vi "output.vi"(8 "error in":errorcluster, 10 "data table in":T1, 11 "OPC UA runtime in":refnum<class "OPC UA Client runtime.lvclass">) -> (0 "error out":errorcluster, 2 "data table out":T1, 3 "OPC UA runtime out":refnum<class "OPC UA Client runtime.lvclass">)   [LabVIEW 2014, in "OPC UA Client runtime.lvclass"]
doc: "Provides an interface for writing data to a module at runtime. While this interface performs no operations, a child should provide an override which may write to any open sessions, references, or interfaces."
uses:
  OPC UA Client runtime.lvclass
  <vilib>/NI/Tag Bus/table/data table.ctl
  OPC UA Client runtime.lvclass/OPC UA Client runtime.ctl
  <vilib>/NI/Tag Bus/table/data polymorphs/read one/read Boolean.vi
  <vilib>/NI/Tag Bus/table/data polymorphs/read one/read I8.vi
  <vilib>/NI/Tag Bus/table/data polymorphs/read one/read U8.vi
  <vilib>/NI/Tag Bus/table/data polymorphs/read one/read I16.vi
  <vilib>/NI/Tag Bus/table/data polymorphs/read one/read U16.vi
  <vilib>/NI/Tag Bus/table/data polymorphs/read one/read I32.vi
  <vilib>/NI/Tag Bus/table/data polymorphs/read one/read U32.vi
  <vilib>/NI/Tag Bus/table/data polymorphs/read one/read I64.vi
  <vilib>/NI/Tag Bus/table/data polymorphs/read one/read U64.vi
  <vilib>/NI/Tag Bus/table/data polymorphs/read one/read Single.vi
  <vilib>/NI/Tag Bus/table/data polymorphs/read one/read Double.vi
  <vilib>/NI/Tag Bus/table/data polymorphs/read one/read String.vi
  <vilib>/NI/Tag Bus/table/data polymorphs/read one/read Array of Boolean.vi
  <vilib>/NI/Tag Bus/table/data polymorphs/read one/read Array of I8.vi
  <vilib>/NI/Tag Bus/table/data polymorphs/read one/read Array of U8.vi
  <vilib>/NI/Tag Bus/table/data polymorphs/read one/read Array of I16.vi
  <vilib>/NI/Tag Bus/table/data polymorphs/read one/read Array of U16.vi
  <vilib>/NI/Tag Bus/table/data polymorphs/read one/read Array of I32.vi
  <vilib>/NI/Tag Bus/table/data polymorphs/read one/read Array of U32.vi
  <vilib>/NI/Tag Bus/table/data polymorphs/read one/read Array of I64.vi
  <vilib>/NI/Tag Bus/table/data polymorphs/read one/read Array of U64.vi
  <vilib>/NI/Tag Bus/table/data polymorphs/read one/read Array of Single.vi
  <vilib>/NI/Tag Bus/table/data polymorphs/read one/read Array of Double.vi
  <vilib>/NI/Tag Bus/table/data polymorphs/read one/read Array of String.vi
  <vilib>/OPCUA/client/Write Bool.vi
  <vilib>/OPCUA/client/Write SByte.vi
  <vilib>/OPCUA/client/Write Byte.vi
  <vilib>/OPCUA/client/Write Int16.vi
  <vilib>/OPCUA/client/Write UInt16.vi
  <vilib>/OPCUA/client/Write Int32.vi
  <vilib>/OPCUA/client/Write UInt32.vi
  <vilib>/OPCUA/client/Write Int64.vi
  <vilib>/OPCUA/client/Write UInt64.vi
  <vilib>/OPCUA/client/Write Float.vi
  <vilib>/OPCUA/client/Write Double.vi
  <vilib>/OPCUA/client/Write String.vi
  <vilib>/OPCUA/client/Write DateTime.vi
  <vilib>/OPCUA/client/Write ByteString.vi
  <vilib>/OPCUA/client/Write Bool Array.vi
  <vilib>/OPCUA/client/Write SByte Array.vi
  <vilib>/OPCUA/client/Write Byte Array.vi
  <vilib>/OPCUA/client/Write Int16 Array.vi
  <vilib>/OPCUA/client/Write UInt16 Array.vi
  <vilib>/OPCUA/client/Write Int32 Array.vi
  <vilib>/OPCUA/client/Write UInt32 Array.vi
  <vilib>/OPCUA/client/Write Int64 Array.vi
  <vilib>/OPCUA/client/Write UInt64 Array.vi
  <vilib>/OPCUA/client/Write Float Array.vi
  <vilib>/OPCUA/client/Write Double Array.vi
  <vilib>/OPCUA/client/Write String Array.vi
  <vilib>/OPCUA/client/Write DateTime Array.vi
  <vilib>/OPCUA/client/Write ByteString Array.vi
  <vilib>/Utility/error.llb/Error Cluster From Error Code.vi
  <vilib>/ErrorRing/Error Ring.xnode
  <vilib>/NI/Tag Bus/table/data table.lvlib
  <vilib>/OPCUA/NI OPC UA Client.lvlib
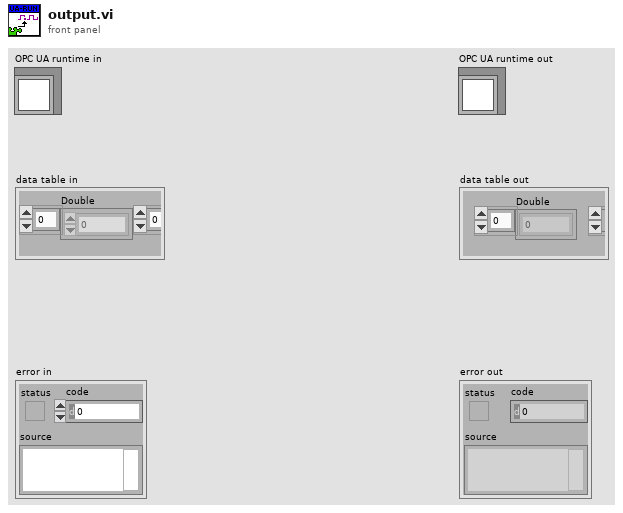
[diagram p1: front panel]
types:
  T1 = typedef "tag bus.lvlib/data table.lvlib/data table.ctl" = cluster{"Double":dbl[], "Single":sgl[], "I64":i64[], "I32":i32[], "I16":i16[], "I8":i8[], "U64":u64[], "U32":u32[], "U16":u16[], "U8":u8[], "Boolean":bool[], "String":string[], "Array of Double":cluster{"DBL Array":dbl[]}[], "Array of Single":cluster{"SGL Array":sgl[]}[], "Array of I64":cluster{"I64 Array":i64[]}[], "Array of I32":cluster{"I32 Array":i32[]}[], "Array of I16":cluster{"I16 Array":i16[]}[], "Array of I8":cluster{"I8 Array":i8[]}[], "Array of U64":cluster{"U64 Array":u64[]}[], "Array of U32":cluster{"U32 Array":u32[]}[], "Array of U16":cluster{"U16 Array":u16[]}[], "Array of U8":cluster{"U8 Array":u8[]}[], "Array of Boolean":cluster{"Boolean Array":bool[]}[], "Array of String":cluster{"String Array":string[]}[]}
  T2 = typedef "tag bus.lvlib/tag descriptor.lvclass/Data Type.ctl" = enum16{"Double", "Single", "I64", "I32", "I16", "I8", "U64", "U32", "U16", "U8", "Boolean", "String", "Array of Double", "Array of Single", "Array of I64", "Array of I32", "Array of I16", "Array of I8", "Array of U64", "Array of U32", "Array of U16", "Array of U8", "Array of Boolean", "Array of String"}
  T3 = typedef "OPC UA Client configuration.lvclass/OPC UA Data Type.ctl" = u16
  T4 = cluster{"DCAF Data Type":T2, "Index":i32, "Node Path":string, "OPC UA Data Type":T3}[]
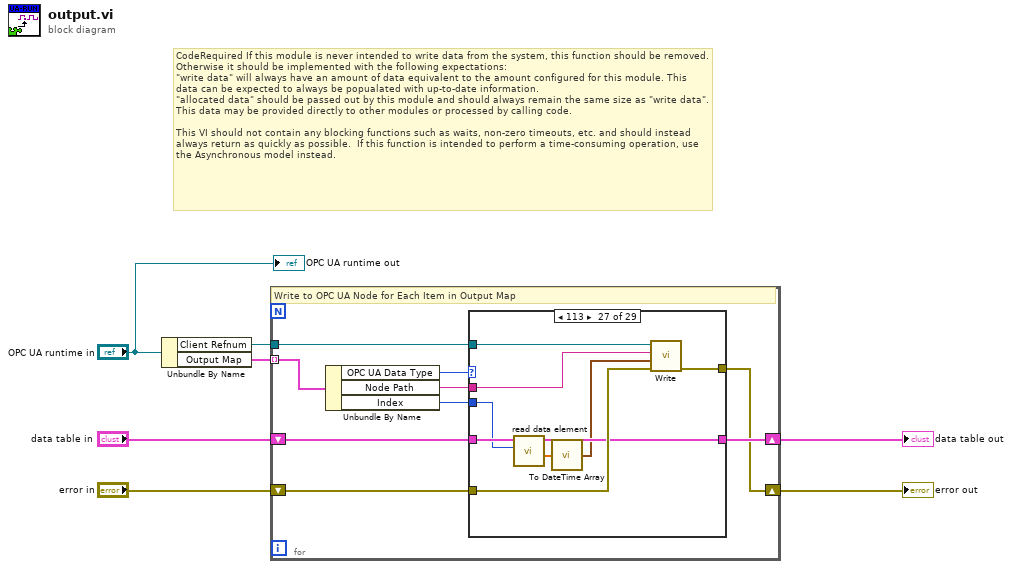
[diagram p0: block diagram]
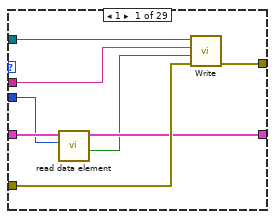
[diagram p2: hidden frame]
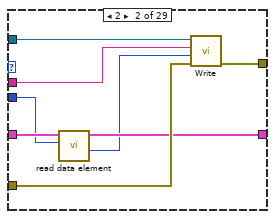
[diagram p3: hidden frame]
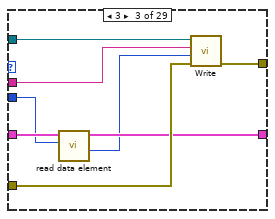
[diagram p4: hidden frame]
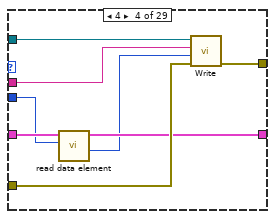
[diagram p5: hidden frame]
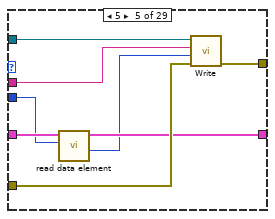
[diagram p6: hidden frame]
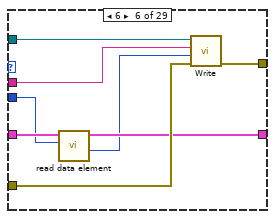
[diagram p7: hidden frame]
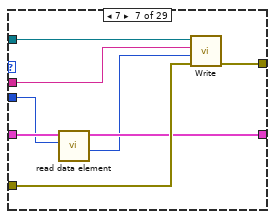
[diagram p8: hidden frame]
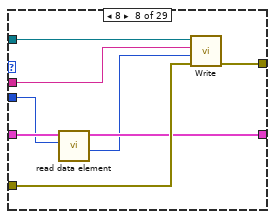
[diagram p9: hidden frame]
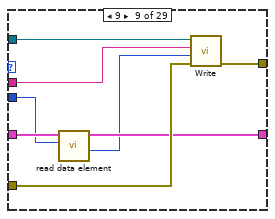
[diagram p10: hidden frame]
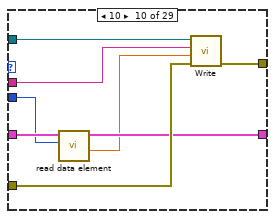
[diagram p11: hidden frame]
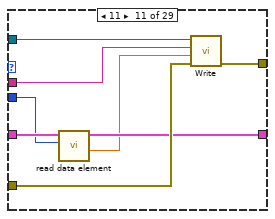
[diagram p12: hidden frame]
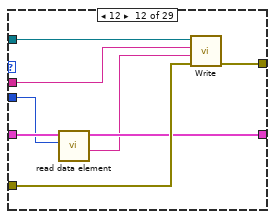
[diagram p13: hidden frame]
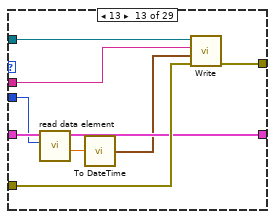
[diagram p14: hidden frame]
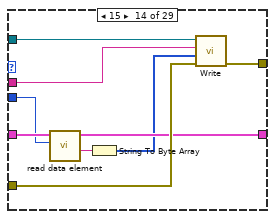
[diagram p15: hidden frame]
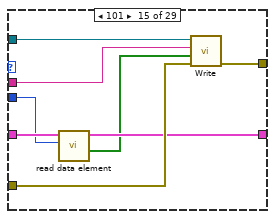
[diagram p16: hidden frame]
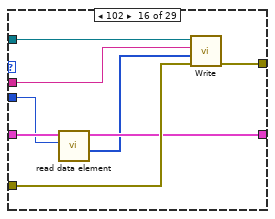
[diagram p17: hidden frame]
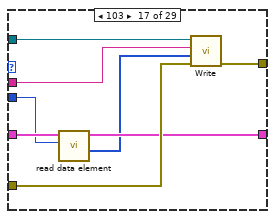
[diagram p18: hidden frame]
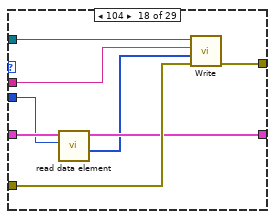
[diagram p19: hidden frame]
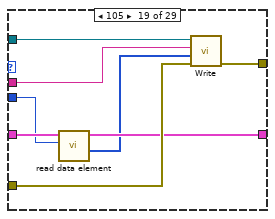
[diagram p20: hidden frame]
diagram:
  # "CodeRequired If this module is never intended to write data from the system, this function should be removed. Otherwise it should be implemented with the following expectations:\n\"write data\" will always have an amount of data equivalent to the amount configured for this module. This data can be expected to always be popualated with up-to-date information.\n\"allocated data\" should be passed out by this module and should always remain the same size as \"write data\". This data may be provided directly to other modules or processed by calling code.\n\nThis VI should not contain any blocking functions such as waits, non-zero timeouts, etc. and should instead always return as quickly as possible.  If this function is intended to perform a time-consuming operation, use the Asynchronous model instead."
  n1 = Unbundle By Name("OPC UA runtime in") -> ("Client Refnum"=w1:refnum<k21>, "Output Map"=w3:T4)
  n2 = for {
    tunnel: w3 -> [w16] mode=indexing
    shift-right: [w10] -> w5
    shift-left: "error in" -> [w12]
    shift-right: [w11] -> w4
    shift-left: "data table in" -> [w14]
    tunnel: w1 -> [w8]
    # "Write to OPC UA Node for Each Item in Output Map"
    n3 = Unbundle By Name(w16) -> ("OPC UA Data Type"=w15:T3, "Node Path"=w9:string, "Index"=w13:i32)
    n4 = case shown="113" w15 {
      tunnel: w14 -> [w24 w32 w40 w48 w56 w64 w72 w80 w88 w96 w104 w112 w121 w130 w138 w146 w154 w162 w170 w178 w186 w194 w202 w210 w218 w226 w235 w244 w247]
      tunnel: w13 -> [w23 w31 w39 w47 w55 w63 w71 w79 w87 w95 w103 w111 w120 w129 w137 w145 w153 w161 w169 w177 w185 w193 w201 w209 w217 w225 w234 w243 _]
      tunnel: w8 -> [w22 w30 w38 w46 w54 w62 w70 w78 w86 w94 w102 w110 w119 w128 w136 w144 w152 w160 w168 w176 w184 w192 w200 w208 w216 w224 w233 w242 _]
      tunnel: w12 -> [w21 w29 w37 w45 w53 w61 w69 w77 w85 w93 w101 w109 w118 w127 w135 w143 w151 w159 w167 w175 w183 w191 w199 w207 w215 w223 w232 w241 _]
      tunnel: [w20 w28 w36 w44 w52 w60 w68 w76 w84 w92 w100 w108 w117 w126 w134 w142 w150 w158 w166 w174 w182 w190 w198 w206 w214 w222 w231 w240 w247] -> w11
      tunnel: [w19 w27 w35 w43 w51 w59 w67 w75 w83 w91 w99 w107 w116 w125 w133 w141 w149 w157 w165 w173 w181 w189 w197 w205 w213 w221 w230 w239 w248] -> w10
      tunnel: w9 -> [w17 w25 w33 w41 w49 w57 w65 w73 w81 w89 w97 w105 w115 w124 w131 w139 w147 w155 w163 w171 w179 w187 w195 w203 w211 w219 w229 w238 _]
      frame 1 {
        n5 = call-poly <vilib>:"read data element.vi"("index"=w23, "data table in"=w24) -> ("value"=w18:bool, "data table out"=w20:T1)  [unwired: 8 in]
        n6 = call-poly <vilib>:"Write.vi"("error in (no error)"=w21, "value"=w18, "node path"=w17, "OPC UA client refnum in"=w22) -> ("error out"=w19:errorcluster)  [unwired: 5 in, 2 out]
      }
      frame 2 {
        n7 = call-poly <vilib>:"read data element.vi"("index"=w31, "data table in"=w32) -> ("value"=w26:i8, "data table out"=w28:T1)  [unwired: 8 in]
        n8 = call-poly <vilib>:"Write.vi"("error in (no error)"=w29, "value"=w26, "node path"=w25, "OPC UA client refnum in"=w30) -> ("error out"=w27:errorcluster)  [unwired: 5 in, 2 out]
      }
      frame 3 {
        n9 = call-poly <vilib>:"read data element.vi"("index"=w39, "data table in"=w40) -> ("value"=w34:u8, "data table out"=w36:T1)  [unwired: 8 in]
        n10 = call-poly <vilib>:"Write.vi"("error in (no error)"=w37, "value"=w34, "node path"=w33, "OPC UA client refnum in"=w38) -> ("error out"=w35:errorcluster)  [unwired: 5 in, 2 out]
      }
      frame 4 {
        n11 = call-poly <vilib>:"read data element.vi"("index"=w47, "data table in"=w48) -> ("value"=w42:i16, "data table out"=w44:T1)  [unwired: 8 in]
        n12 = call-poly <vilib>:"Write.vi"("error in (no error)"=w45, "value"=w42, "node path"=w41, "OPC UA client refnum in"=w46) -> ("error out"=w43:errorcluster)  [unwired: 5 in, 2 out]
      }
      frame 5 {
        n13 = call-poly <vilib>:"read data element.vi"("index"=w55, "data table in"=w56) -> ("value"=w50:u16, "data table out"=w52:T1)  [unwired: 8 in]
        n14 = call-poly <vilib>:"Write.vi"("error in (no error)"=w53, "value"=w50, "node path"=w49, "OPC UA client refnum in"=w54) -> ("error out"=w51:errorcluster)  [unwired: 5 in, 2 out]
      }
      frame 6 {
        n15 = call-poly <vilib>:"read data element.vi"("index"=w63, "data table in"=w64) -> ("value"=w58:i32, "data table out"=w60:T1)  [unwired: 8 in]
        n16 = call-poly <vilib>:"Write.vi"("error in (no error)"=w61, "value"=w58, "node path"=w57, "OPC UA client refnum in"=w62) -> ("error out"=w59:errorcluster)  [unwired: 5 in, 2 out]
      }
      frame 7 {
        n17 = call-poly <vilib>:"read data element.vi"("index"=w71, "data table in"=w72) -> ("value"=w66:u32, "data table out"=w68:T1)  [unwired: 8 in]
        n18 = call-poly <vilib>:"Write.vi"("error in (no error)"=w69, "value"=w66, "node path"=w65, "OPC UA client refnum in"=w70) -> ("error out"=w67:errorcluster)  [unwired: 5 in, 2 out]
      }
      frame 8 {
        n19 = call-poly <vilib>:"read data element.vi"("index"=w79, "data table in"=w80) -> ("value"=w74:i64, "data table out"=w76:T1)  [unwired: 8 in]
        n20 = call-poly <vilib>:"Write.vi"("error in (no error)"=w77, "value"=w74, "node path"=w73, "OPC UA client refnum in"=w78) -> ("error out"=w75:errorcluster)  [unwired: 5 in, 2 out]
      }
      frame 9 {
        n21 = call-poly <vilib>:"read data element.vi"("index"=w87, "data table in"=w88) -> ("value"=w82:u64, "data table out"=w84:T1)  [unwired: 8 in]
        n22 = call-poly <vilib>:"Write.vi"("error in (no error)"=w85, "value"=w82, "node path"=w81, "OPC UA client refnum in"=w86) -> ("error out"=w83:errorcluster)  [unwired: 5 in, 2 out]
      }
      frame 10 {
        n23 = call-poly <vilib>:"read data element.vi"("index"=w95, "data table in"=w96) -> ("value"=w90:sgl, "data table out"=w92:T1)  [unwired: 8 in]
        n24 = call-poly <vilib>:"Write.vi"("error in (no error)"=w93, "value"=w90, "node path"=w89, "OPC UA client refnum in"=w94) -> ("error out"=w91:errorcluster)  [unwired: 5 in, 2 out]
      }
      frame 11 {
        n25 = call-poly <vilib>:"read data element.vi"("index"=w103, "data table in"=w104) -> ("value"=w98:dbl, "data table out"=w100:T1)  [unwired: 8 in]
        n26 = call-poly <vilib>:"Write.vi"("error in (no error)"=w101, "value"=w98, "node path"=w97, "OPC UA client refnum in"=w102) -> ("error out"=w99:errorcluster)  [unwired: 5 in, 2 out]
      }
      frame 12 {
        n27 = call-poly <vilib>:"read data element.vi"("index"=w111, "data table in"=w112) -> ("value"=w106:string, "data table out"=w108:T1)  [unwired: 8 in]
        n28 = call-poly <vilib>:"Write.vi"("error in (no error)"=w109, "value"=w106, "node path"=w105, "OPC UA client refnum in"=w110) -> ("error out"=w107:errorcluster)  [unwired: 5 in, 2 out]
      }
      frame 13 {
        n29 = call-poly <vilib>:"read data element.vi"("index"=w120, "data table in"=w121) -> ("value"=w114:dbl, "data table out"=w117:T1)  [unwired: 8 in]
        n30 = call "To DateTime.vi"("Formatted DateTime"=w114) -> ("Time Stamp"=w113:timestamp)
        n31 = call-poly <vilib>:"Write.vi"("error in (no error)"=w118, "value"=w113, "node path"=w115, "OPC UA client refnum in"=w119) -> ("error out"=w116:errorcluster)  [unwired: 5 in, 2 out]
      }
      frame 15 {
        n32 = call-poly <vilib>:"read data element.vi"("index"=w129, "data table in"=w130) -> ("value"=w123:string, "data table out"=w126:T1)  [unwired: 8 in]
        n33 = String To Byte Array(string=w123) -> (unsigned byte array=w122:u8[])
        n34 = call-poly <vilib>:"Write.vi"("error in (no error)"=w127, "value"=w122, "node path"=w124, "OPC UA client refnum in"=w128) -> ("error out"=w125:errorcluster)  [unwired: 5 in, 2 out]
      }
      frame 101 {
        n35 = call-poly <vilib>:"read data element.vi"("index"=w137, "data table in"=w138) -> ("value"=w132:bool[], "data table out"=w134:T1)  [unwired: 8 in]
        n36 = call-poly <vilib>:"Write.vi"("error in (no error)"=w135, "value"=w132, "node path"=w131, "OPC UA client refnum in"=w136) -> ("error out"=w133:errorcluster)  [unwired: 5 in, 2 out]
      }
      frame 102 {
        n37 = call-poly <vilib>:"read data element.vi"("index"=w145, "data table in"=w146) -> ("value"=w140:i8[], "data table out"=w142:T1)  [unwired: 8 in]
        n38 = call-poly <vilib>:"Write.vi"("error in (no error)"=w143, "value"=w140, "node path"=w139, "OPC UA client refnum in"=w144) -> ("error out"=w141:errorcluster)  [unwired: 5 in, 2 out]
      }
      frame 103 {
        n39 = call-poly <vilib>:"read data element.vi"("index"=w153, "data table in"=w154) -> ("value"=w148:u8[], "data table out"=w150:T1)  [unwired: 8 in]
        n40 = call-poly <vilib>:"Write.vi"("error in (no error)"=w151, "value"=w148, "node path"=w147, "OPC UA client refnum in"=w152) -> ("error out"=w149:errorcluster)  [unwired: 5 in, 2 out]
      }
      frame 104 {
        n41 = call-poly <vilib>:"read data element.vi"("index"=w161, "data table in"=w162) -> ("value"=w156:i16[], "data table out"=w158:T1)  [unwired: 8 in]
        n42 = call-poly <vilib>:"Write.vi"("error in (no error)"=w159, "value"=w156, "node path"=w155, "OPC UA client refnum in"=w160) -> ("error out"=w157:errorcluster)  [unwired: 5 in, 2 out]
      }
      frame 105 {
        n43 = call-poly <vilib>:"read data element.vi"("index"=w169, "data table in"=w170) -> ("value"=w164:u16[], "data table out"=w166:T1)  [unwired: 8 in]
        n44 = call-poly <vilib>:"Write.vi"("error in (no error)"=w167, "value"=w164, "node path"=w163, "OPC UA client refnum in"=w168) -> ("error out"=w165:errorcluster)  [unwired: 5 in, 2 out]
      }
      frame 106 {
        n45 = call-poly <vilib>:"read data element.vi"("index"=w177, "data table in"=w178) -> ("value"=w172:i32[], "data table out"=w174:T1)  [unwired: 8 in]
        n46 = call-poly <vilib>:"Write.vi"("error in (no error)"=w175, "value"=w172, "node path"=w171, "OPC UA client refnum in"=w176) -> ("error out"=w173:errorcluster)  [unwired: 5 in, 2 out]
      }
      frame 107 {
        n47 = call-poly <vilib>:"read data element.vi"("index"=w185, "data table in"=w186) -> ("value"=w180:u32[], "data table out"=w182:T1)  [unwired: 8 in]
        n48 = call-poly <vilib>:"Write.vi"("error in (no error)"=w183, "value"=w180, "node path"=w179, "OPC UA client refnum in"=w184) -> ("error out"=w181:errorcluster)  [unwired: 5 in, 2 out]
      }
      frame 108 {
        n49 = call-poly <vilib>:"read data element.vi"("index"=w193, "data table in"=w194) -> ("value"=w188:i64[], "data table out"=w190:T1)  [unwired: 8 in]
        n50 = call-poly <vilib>:"Write.vi"("error in (no error)"=w191, "value"=w188, "node path"=w187, "OPC UA client refnum in"=w192) -> ("error out"=w189:errorcluster)  [unwired: 5 in, 2 out]
      }
      frame 109 {
        n51 = call-poly <vilib>:"read data element.vi"("index"=w201, "data table in"=w202) -> ("value"=w196:u64[], "data table out"=w198:T1)  [unwired: 8 in]
        n52 = call-poly <vilib>:"Write.vi"("error in (no error)"=w199, "value"=w196, "node path"=w195, "OPC UA client refnum in"=w200) -> ("error out"=w197:errorcluster)  [unwired: 5 in, 2 out]
      }
      frame 110 {
        n53 = call-poly <vilib>:"read data element.vi"("index"=w209, "data table in"=w210) -> ("value"=w204:sgl[], "data table out"=w206:T1)  [unwired: 8 in]
        n54 = call-poly <vilib>:"Write.vi"("error in (no error)"=w207, "value"=w204, "node path"=w203, "OPC UA client refnum in"=w208) -> ("error out"=w205:errorcluster)  [unwired: 5 in, 2 out]
      }
      frame 111 {
        n55 = call-poly <vilib>:"read data element.vi"("index"=w217, "data table in"=w218) -> ("value"=w212:dbl[], "data table out"=w214:T1)  [unwired: 8 in]
        n56 = call-poly <vilib>:"Write.vi"("error in (no error)"=w215, "value"=w212, "node path"=w211, "OPC UA client refnum in"=w216) -> ("error out"=w213:errorcluster)  [unwired: 5 in, 2 out]
      }
      frame 112 {
        n57 = call-poly <vilib>:"read data element.vi"("index"=w225, "data table in"=w226) -> ("value"=w220:string[], "data table out"=w222:T1)  [unwired: 8 in]
        n58 = call-poly <vilib>:"Write.vi"("error in (no error)"=w223, "value"=w220, "node path"=w219, "OPC UA client refnum in"=w224) -> ("error out"=w221:errorcluster)  [unwired: 5 in, 2 out]
      }
      frame 113 {
        n59 = call-poly <vilib>:"read data element.vi"("index"=w234, "data table in"=w235) -> ("value"=w228:dbl[], "data table out"=w231:T1)  [unwired: 8 in]
        n60 = call "To DateTime Array.vi"("Formatted DateTime Array"=w228) -> ("DateTime Array"=w227:timestamp[])
        n61 = call-poly <vilib>:"Write.vi"("error in (no error)"=w232, "value"=w227, "node path"=w229, "OPC UA client refnum in"=w233) -> ("error out"=w230:errorcluster)  [unwired: 5 in, 2 out]
      }
      frame 115 {
        n62 = call-poly <vilib>:"read data element.vi"("index"=w243, "data table in"=w244) -> ("value"=w237:string[], "data table out"=w240:T1)  [unwired: 8 in]
        n63 = for {
          tunnel: w237 -> [w246] mode=indexing
          tunnel: [w245] -> w236 mode=indexing
          n64 = String To Byte Array(string=w246) -> (unsigned byte array=w245:u8[])
        }
        n65 = call-poly <vilib>:"Write.vi"("error in (no error)"=w241, "value"=w236, "node path"=w238, "OPC UA client refnum in"=w242) -> ("error out"=w239:errorcluster)  [unwired: 5 in, 2 out]
      }
      frame 0, Default {
        # "invalid data type, throw error"
        n66 = xnode "Error Ring"() -> ("error out"=w248:errorcluster)
      }
    }
  }
  "error out" <- w5
  "data table out" <- w4
  "OPC UA runtime out" <- "OPC UA runtime in"
